vi "Get Initialize Hot And Cold Source Unit.vi"(8 "error in (no error)":errorcluster, 11 "Abstract Initialize Hot And Cold Source Unit Msg in":refnum<class "Abstract Initialize Hot And Cold Source Unit Msg.lvclass">) -> (0 "error out":errorcluster, 2 "Initialize Hot And Cold Source Unit":bool, 3 "Abstract Initialize Hot And Cold Source Unit Msg out":refnum<class "Abstract Initialize Hot And Cold Source Unit Msg.lvclass">)   [LabVIEW 2013, in "Hot And Cold Source Unit Model.lvlib" / "Abstract Initialize Hot And Cold Source Unit Msg.lvclass"]
uses:
  Abstract Initialize Hot And Cold Source Unit Msg.lvclass
  Abstract Initialize Hot And Cold Source Unit Msg.lvclass/Abstract Initialize Hot And Cold Source Unit Msg.ctl
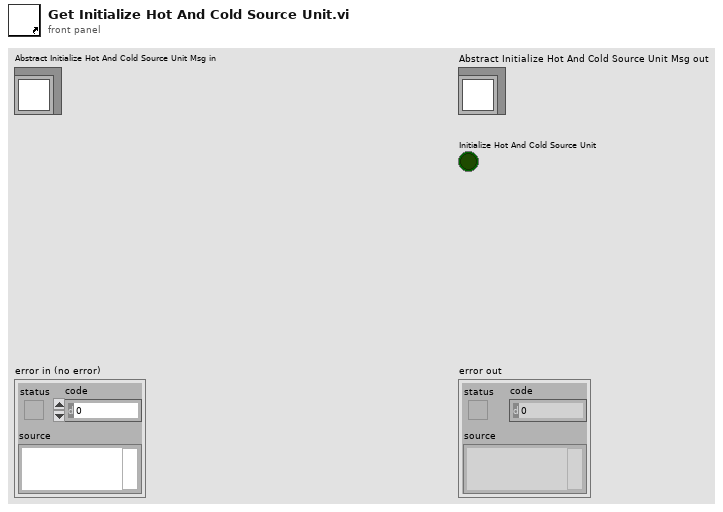
[diagram p1: front panel]
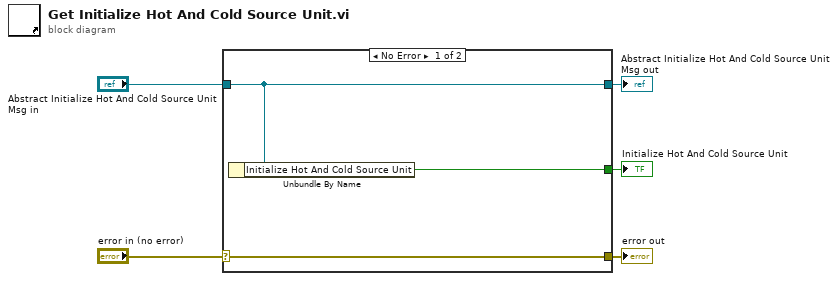
[diagram p0: block diagram]
diagram:
  n1 = case shown="No Error" "error in (no error)" {
    selector: "error in (no error)" -> [w8 w9]
    tunnel: [w8 w9] -> w4
    tunnel: [w7 w10] -> w2
    tunnel: "Abstract Initialize Hot And Cold Source Unit Msg in" -> [w7 w10]
    tunnel: [w6 _] -> w1
    frame No Error {
      n2 = Unbundle By Name(w7) -> ("Initialize Hot And Cold Source Unit"=w6:bool)
    }
    frame Error {
    }
  }
  "error out" <- w4
  "Abstract Initialize Hot And Cold Source Unit Msg out" <- w2
  "Initialize Hot And Cold Source Unit" <- w1
